vi "Copy Client Template Library.vi"(8 "error in":errorcluster, 10 "client name":string, 11 "project ref":refnum<vi>) -> (0 "error out":errorcluster, 2 "measure vi refnum":refnum<vi>, 3 "project ref out":refnum<vi>)   [LabVIEW 2021, in "MeasurementClient Editor.lvlib"]
uses:
  MeasurementClient Editor.lvlib
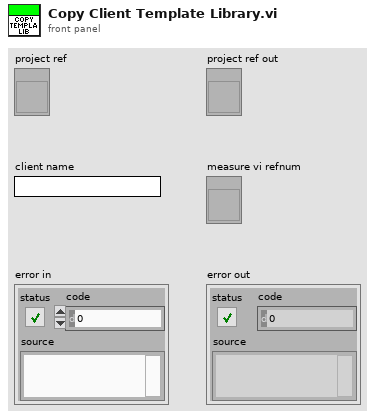
[diagram p1: front panel]
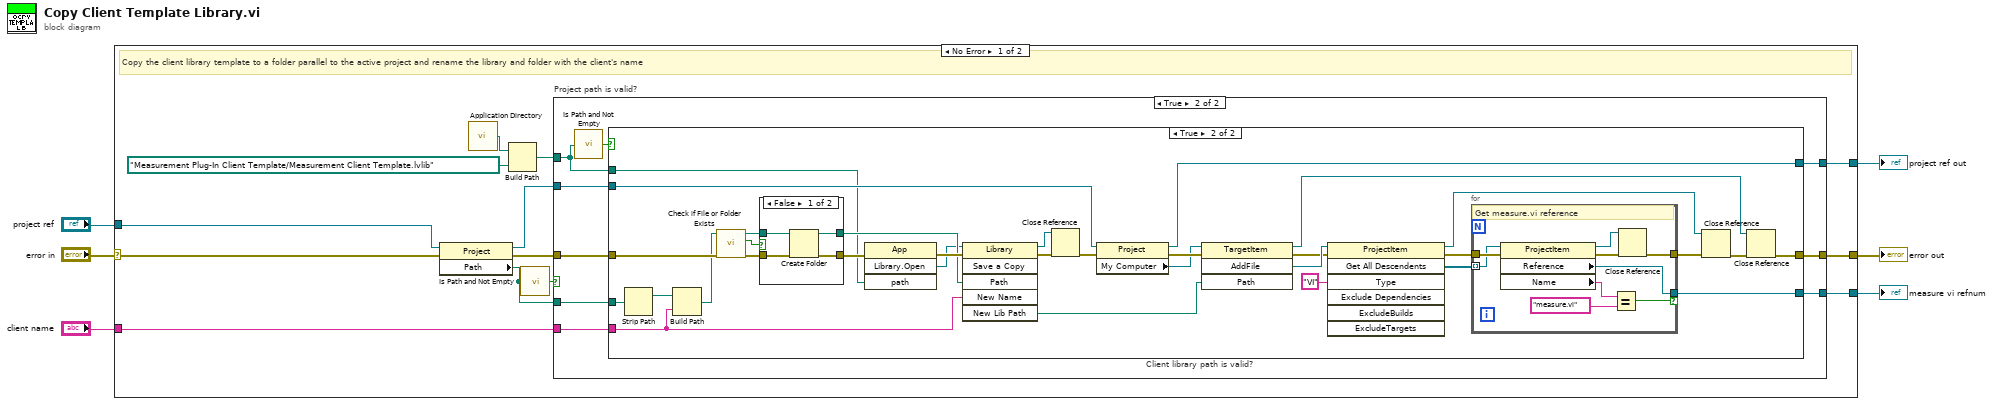
[diagram p0: block diagram]
diagram:
  n1 = case shown="No Error" "error in" {
    selector: "error in" -> [w17 w81]
    tunnel: "project ref" -> [w19 w80]
    tunnel: "client name" -> [w13 _]
    tunnel: [w9 w81] -> w3
    tunnel: [w8 w80] -> w2
    tunnel: [w7 _] -> w1
    frame No Error {
      # "Copy the client library template to a folder parallel to the active project and rename the library and folder with the client's name"
      n2 = property class="Project"(reference=w19, error in=w17) -> (reference out=w10:refnum<vi>, error out=w18:errorcluster, "Path"=w14:path)
      n3 = call <vilib>:"Application Directory.vi"() -> ("Application Directory"=w15:path)
      n4 = Build Path(base path=w15, name or relative path=path "Measurement Plug-In Client Template/Measurement Client Template.lvlib") -> (appended path=w12:path)
      n5 = call <vilib>:"Is Path and Not Empty.vi"("path"=w14) -> ("Is Path and Not Empty?"=w16:bool)  [unwired: 4 in]
      n6 = case "Project path is valid?" shown="True" w16 {
        tunnel: w18 -> [w21 w30]
        tunnel: w12 -> [_ w23]
        tunnel: w14 -> [_ w29]
        tunnel: w13 -> [_ w28]
        tunnel: w10 -> [w20 w27]
        tunnel: [w21 w26] -> w9
        tunnel: [w20 w25] -> w8
        tunnel: [_ w24] -> w7
        frame False {
        }
        frame True {
          n7 = call <vilib>:"Is Path and Not Empty.vi"("path"=w23) -> ("Is Path and Not Empty?"=w22:bool)  [unwired: 4 in]
          n8 = case "Client library path is valid?" shown="True" w22 {
            tunnel: w30 -> [w32 w64]
            tunnel: w29 -> [_ w62]
            tunnel: w28 -> [_ w54]
            tunnel: w27 -> [w31 w52]
            tunnel: [w32 w38] -> w26
            tunnel: [w31 w36] -> w25
            tunnel: [_ w35] -> w24
            tunnel: w23 -> [_ w34]
            frame False {
            }
            frame True {
              n9 = Strip Path(path=w62) -> (stripped path=w61:path)  [unwired: 1 out]
              n10 = Build Path(base path=w61, name or relative path=w54) -> (appended path=w60:path)
              n11 = call <vilib>:"Check if File or Folder Exists.vi"("error in (no error)"=w64, "path"=w60) -> ("error out"=w59:errorcluster, "file or folder exists?"=w58:bool, "dup path"=w57:path)  [unwired: 7 in]
              n12 = case shown="False" w58 {
                tunnel: w59 -> [w77 w78]
                tunnel: w57 -> [w76 w79]
                tunnel: [w75 w78] -> w55
                tunnel: [w74 w79] -> w56
                frame False {
                  n13 = Create Folder(path (use dialog)=w76, error in=w77) -> (created path=w74:path, error out=w75:errorcluster)  [unwired: 1 in, 1 out]
                }
                frame True {
                }
              }
              n14 = invoke class="App" method="Library.Open"(error in=w55, "path"=w34) -> (error out=w63:errorcluster, "Open Library"=w53:refnum<vi>)  [unwired: 2 in, 2 out]
              n15 = invoke class="Library" method="Save a Copy"(reference=w53, error in=w63, "Path"=w56, "New Name"=w54) -> (reference out=w49:refnum<vi>, error out=w50:errorcluster, "New Lib Path"=w47:path)  [unwired: 2 in, 3 out]
              n16 = Close Reference(reference=w49, error in (no error)=w50) -> (error out=w51:errorcluster)
              n17 = property class="Project"(reference=w52, error in=w51) -> (reference out=w36:refnum<vi>, error out=w48:errorcluster, "My Computer"=w37:refnum<vi>)
              n18 = invoke class="TargetItem" method="AddFile"(reference=w37, error in=w48, "Path"=w47) -> (reference out=w40:refnum<vi>, error out=w45:errorcluster, "AddFile"=w46:refnum<vi>)  [unwired: 1 in, 1 out]
              n19 = invoke class="ProjectItem" method="Get All Descendents"(reference=w46, error in=w45, "Type"="VI") -> (reference out=w39:refnum<vi>, error out=w43:errorcluster, "All Descendents"=w42:refnum<vi>[])  [unwired: 4 in, 4 out]
              n20 = for {
                tunnel: w43 -> [w73]
                tunnel: w42 -> [w72] mode=indexing
                tunnel: [w69] -> w35 if=w68
                tunnel: [w65] -> w33
                # "Get measure.vi reference"
                n21 = property class="ProjectItem"(reference=w72, error in=w73) -> (reference out=w71:refnum<vi>, error out=w67:errorcluster, "Reference"=w69:refnum<vi>, "Name"=w70:string)
                n22 = Equal?(x=w70, y="measure.vi") -> (x = y?=w68:bool)
                n23 = Close Reference(reference=w71, error in (no error)=w67) -> (error out=w65:errorcluster)
              }
              n24 = Close Reference(reference=w39, error in (no error)=w33) -> (error out=w41:errorcluster)
              n25 = Close Reference(reference=w40, error in (no error)=w41) -> (error out=w38:errorcluster)
            }
          }
        }
      }
    }
    frame Error {
      # "Pass"
    }
  }
  "error out" <- w3
  "project ref out" <- w2
  "measure vi refnum" <- w1
